vi "Get Class List from Folder.vi"(8 "error in (no error)":errorcluster, 11 "Folder Path":path) -> (0 "error out":errorcluster, 3 "Class List[]":path[](array[path]))   [LabVIEW 2016, in "SLL Class.lvlib"]
uses:
  SLL Class.lvlib
  <vilib>/Utility/LVLibp/NI_PackedLibraryUtility.lvlib
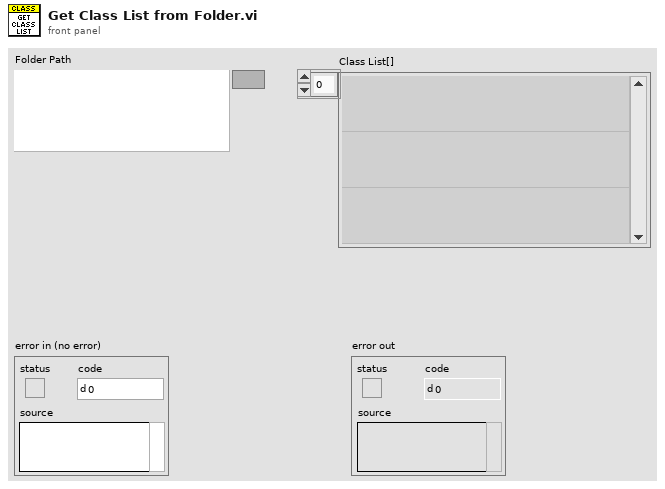
[diagram p1: front panel]
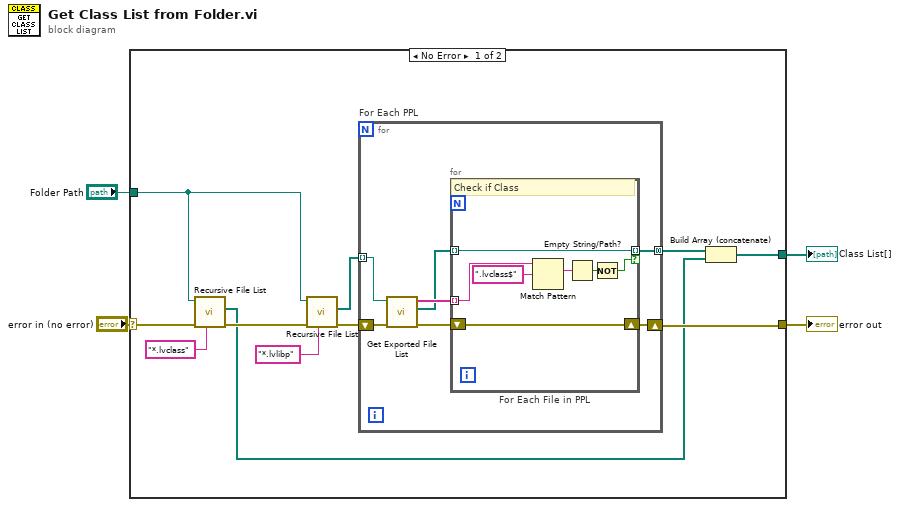
[diagram p0: block diagram]
diagram:
  n1 = case shown="No Error" "error in (no error)" {
    selector: "error in (no error)" -> [w15 w30]
    tunnel: [w8 w30] -> w3
    tunnel: "Folder Path" -> [w12 _]
    tunnel: [w5 _] -> w1
    frame No Error {
      n2 = call <vilib>:"Recursive File List.vi"("pattern"="*.lvclass", "error in (no error)"=w15, "Folder Path"=w12) -> ("error out"=w13:errorcluster, "All Files in Dir"=w7:path[])  [unwired: 4 in, 3 out]
      n3 = call <vilib>:"Recursive File List.vi"("pattern"="*.lvlibp", "error in (no error)"=w13, "Folder Path"=w12) -> ("error out"=w10:errorcluster, "All Files in Dir"=w9:path[])  [unwired: 4 in, 3 out]
      n4 = for "For Each PPL" {
        tunnel: w9 -> [w21] mode=indexing
        shift-right: [w17] -> w8
        shift-left: w10 -> [w22]
        tunnel: [w16] -> w6 mode=concatenating
        n5 = call <vilib>:"Get Exported File List.vi"("error in (no error)"=w22, "packed library path"=w21) -> ("error out"=w20:errorcluster, "paths"=w18:path[], "qualified names"=w19:string[])  [unwired: 7 in]
        n6 = for "For Each File in PPL" {
          tunnel: w19 -> [w29] mode=indexing
          tunnel: w18 -> [w25] mode=indexing
          tunnel: [w25] -> w16 mode=indexing if=w23
          shift-right: [w24] -> w17
          shift-left: w20 -> [w24]
          # "Check if Class"
          n7 = Match Pattern(string=w29, regular expression=".lvclass$") -> (match substring=w27:string)  [unwired: 1 in, 3 out]
          n8 = Empty String/Path?(string/path=w27) -> (empty?=w26:bool)
          n9 = Not(x=w26) -> (.not. x?=w23:bool)
        }
      }
      n10 = Build Array (concatenate)(w6, w7) -> (w5:path[])
    }
    frame Error {
    }
  }
  "error out" <- w3
  "Class List[]" <- w1
